vi "ImplModelFollow_GetU.vi"(11 "in IMPLICIT_MODEL_FOLLOWER":T2) -> (3 "U":T1)   [LabVIEW 2019, in "Trajectory_Library.lvlib"]
doc: "Create implicit model follower\n\nInputs:\n - A < states, states > -- Continuous system matrix of the plant being controlled.\n - B < states, inputs > -- Continuous input matrix of the plant being controlled.\n - A_Ref < states, states > -- Continuous system matrix whose dymanics should be followed.\n - B_Ref < states, inputs > -- Continuous input matrix x whose dymanics should be followed.\n\nOutputs:\n - Error -- If TRUE, an error occured."
uses:
  Trajectory_Library.lvlib
  TypeDef/IMPLICIT_MODEL_FOLLOWER.ctl
  <vilib>/Analysis/Matrix/Datatypes/RealMatrix.ctl
  <vilib>/Analysis/Matrix/NI_Matrix.lvlib
panel:
  # "<States,States>"
  # "<States,Inputs>"
  # "<Inputs,1>"
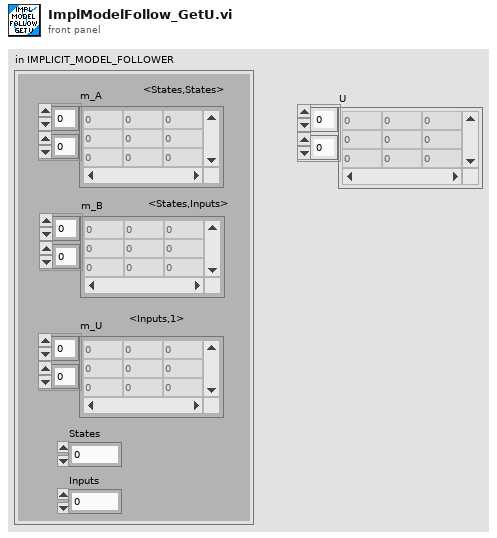
[diagram p1: front panel]
types:
  T1 = typedef "NI_Matrix.lvlib/RealMatrix.ctl" = dbl[][]
  T2 = typedef "Trajectory_Library.lvlib/IMPLICIT_MODEL_FOLLOWER.ctl" = cluster{"m_A":T1, "m_B":T1, "m_U":T1, "States":i32, "Inputs":i32}
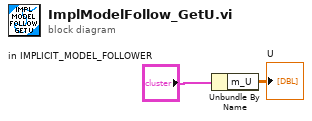
[diagram p0: block diagram]
diagram:
  n1 = Unbundle By Name("in IMPLICIT_MODEL_FOLLOWER") -> ("m_U"=→"U":T1)
